vi "Set Cycle Time.vi"(8 "error in (no error)":errorcluster, 10 "cycle time":u32=1000, 11 "Device in":refnum<class "Device.lvclass">) -> (0 "error out":errorcluster, 3 "Device out":refnum<class "Device.lvclass">)   [LabVIEW 2023, in "Device.lvlib" / "Device.lvclass"]
uses:
  Device.lvclass
  Device.lvclass/Device.ctl
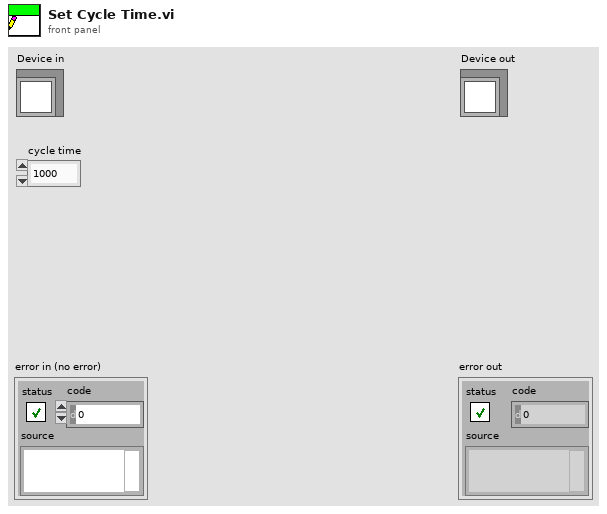
[diagram p1: front panel]
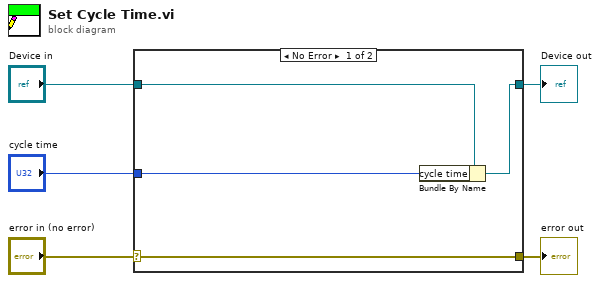
[diagram p0: block diagram]
diagram:
  n1 = case shown="No Error" "error in (no error)" {
    selector: "error in (no error)" -> [w9 w10]
    tunnel: [w9 w10] -> w4
    tunnel: [w7 w11] -> w2
    tunnel: "Device in" -> [w8 w11]
    tunnel: "cycle time" -> [w6 _]
    frame No Error {
      n2 = Bundle By Name(cluster=w8, "cycle time"=w6) -> (w7:refnum<class "Device.lvclass">)
    }
    frame Error {
    }
  }
  "error out" <- w4
  "Device out" <- w2
